vi "GettingStarted_RealSignals.vi"() -> ()   [LabVIEW 2009]
uses:
  <vilib>/imath/engines/lvmath2/RunTimeEngine/ErrorHandling/NIMS_Finalize Error.vi
  <vilib>/imath/engines/lvmath2/RunTimeEngine/Parser/MC_Version.vi
  <vilib>/imath/engines/lvmath2/RunTimeEngine/NodeEndStatement/NIMS_NodeEndStatement_Output.vi
  <instcachedir>/0/NIMS_NodeEndStatement_Output_53EC0D466D134D7ABD903AC30B43404B.lvgen/NIMS_NodeEndStatement_Output_53EC0D466D134D7ABD903AC30B43404B_001.vi
  <vilib>/imath/engines/lvmath2/RunTimeEngine/RangeToken/NIMS_Range.vi
  <instcachedir>/0/NIMS_Range_08574DECC23E450FAF0AC0BC39E6BEA7.lvgen/NIMS_Range_08574DECC23E450FAF0AC0BC39E6BEA7_001.vi
  <vilib>/imathl/engines/lvmath/Functions/Error Handling/Create Error.vi
  <vilib>/imath/engines/lvmath/Functions/Error Handling/MC_Error Cluster From Error Code.vi
  <vilib>/imath/engines/lvmath2/RunTimeEngine/BuiltInFunctions/rand/NIMS_rand(1,I32).vi
  <vilib>/imath/engines/lvmath/Functions/Error Handling/MergeErrorsWrapper.vi
  <vilib>/imath/engines/lvmath2/RunTimeEngine/BuiltInFunctions/abs/NIMS_abs(signed).vi
  <instcachedir>/0/NIMS_abs(signed)_C4FCB8E6058B49B797C7C8D53CA5F6EC.lvgen/NIMS_abs(signed)_C4FCB8E6058B49B797C7C8D53CA5F6EC_000.vi
  <vilib>/imath/engines/lvmath2/RunTimeEngine/BuiltInFunctions/fft/NIMS_fft(GV).vi
  <instcachedir>/0/NIMS_fft(GV)_4C6467FC22F84E4BA42517A07EF978B0.lvgen/NIMS_fft(GV)_4C6467FC22F84E4BA42517A07EF978B0_001.vi
  <vilib>/imath/engines/lvmath2/RunTimeEngine/ArithmeticOperatorToken/NIMS_ArithmeticOperator_plus.vi
  <instcachedir>/0/NIMS_ArithmeticOperator_plus_48B9519178ED42D7840F01273E784BFE.lvgen/NIMS_ArithmeticOperator_plus_48B9519178ED42D7840F01273E784BFE_000.vi
panel:
  in  "Spur Level (V)":dbl=0.001
  in  "Noise Level (V)":dbl(slide)=0.00024489795918367346 scale=0.0..0.001
  in  "Tab Control":T1(tab)=enum."Noise & Signal + Spur"
  out "x":dbl[](graph)=[0.0, 1.0, 2.0, 3.0, 4.0, 5.0, 6.0, 7.0, 8.0, 9.0, 10.0, 11.0, 12.0, 13.0, 14.0, 15.0, 16.0, 17.0, 18.0, 19.0, 20.0, 21.0, 22.0, 23.0, 24.0, 25.0, 26.0, 27.0, 28.0, 29.0, 30.0, 31.0, 32.0, 33.0, 34.0, 35.0, 36.0, 37.0, 38.0, 39.0, 40.0, 41.0, 42.0, 43.0, 44.0, 45.0, 46.0, 47.0, 48.0, 49.0, 50.0, 51.0, 52.0, 53.0, 54.0, 55.0, 56.0, 57.0, 58.0, 59.0, 60.0, 61.0, 62.0, 63.0]
  out "signal (Time Domain)":dbl[](graph)=[1.0, 0.9951847266721969, 0.9807852804032304, 0.9569403357322088, 0.9238795325112867, 0.881921264348355, 0.8314696123025452, 0.773010453362737, 0.7071067811865476, 0.6343932841636455, 0.5555702330196023, 0.4713967368259978, 0.38268343236508984, 0.29028467725446233, 0.19509032201612833, 0.09801714032956077, 6.123031769111886e-17, -0.09801714032956065, -0.1950903220161282, -0.29028467725446216, -0.3826834323650897, -0.4713967368259977, -0.555570233019602, -0.6343932841636454, -0.7071067811865475, -0.773010453362737, -0.8314696123025453, -0.8819212643483549, -0.9238795325112867, -0.9569403357322088, -0.9807852804032304, -0.9951847266721968, -1.0, -0.9951847266721969, -0.9807852804032304, -0.9569403357322089, -0.9238795325112868, -0.881921264348355, -0.8314696123025455, -0.7730104533627371, -0.7071067811865477, -0.6343932841636459, -0.5555702330196022, -0.47139673682599786, -0.38268343236509034, -0.29028467725446244, -0.19509032201612866, -0.09801714032956045, -1.836909530733566e-16, 0.09801714032956009, 0.1950903220161283, 0.29028467725446205, 0.38268343236509, 0.4713967368259976, 0.5555702330196018, 0.6343932841636456, 0.7071067811865474, 0.7730104533627367, 0.8314696123025452, 0.8819212643483548, 0.9238795325112865, 0.9569403357322088, 0.9807852804032303, 0.9951847266721969]
  out "noise (Time Domain)":dbl[](graph)=[0.00017345388847732183, 9.384721690440629e-05, 0.00021325506107333988, 9.033739461556139e-05, 8.225115957588394e-05, 0.00022899374260867145, 0.00017108200961533386, 4.3499454064839606e-05, 4.216960210159472e-05, 5.300855810985709e-05, 0.00022634691048571397, 4.142058298539253e-05, 0.00010698946173820982, 0.00017919168575125506, 0.000228746962935423, 0.00016811831847637424, 0.000149018054221302, 8.26228389545729e-05, 5.108267442002953e-05, 0.00022921494428844056, 0.00021666900139901673, 0.00018958850216650077, 6.182126932943757e-05, 0.0001013976231695041, 8.718964914935843e-05, 0.00013324340118243882, 0.0002384798798628175, 6.321954061707498e-05, 5.9741047834780797e-05, 4.5206442745249866e-05, 4.30637612234021e-05, 3.932217315793377e-05, 6.520083152831608e-05, 0.00023048966084202114, 3.048846374611175e-05, 4.528958373625526e-05, 4.425462708597921e-05, 0.00020517114908387817, 0.00014397299183518258, 0.00020960760994048083, 0.0001678937735573273, 0.00017945446738414523, 0.00014919763515730956, 0.00022121817515546554, 0.00010548017003027697, 0.00018691125297748206, 0.00014788947043336631, 5.466160312999556e-05, 1.0369681325846585e-05, 5.203831786508366e-05, 6.491243230331916e-05, 0.000236582660093371, 0.0001363150245849827, 4.065564633537551e-05, 7.924747061934878e-05, 0.00022262559485221323, 0.00011413358700753988, 3.354305722250164e-05, 0.00018280271967387516, 0.00022227396517330978, 0.0002219588013856892, 0.00021367238122965265, 2.8128510108291296e-05, 0.0002404575102916334]
  out "Signal+noise (Time Domain)":dbl[](graph)=[1.0001734538884772, 0.9952785738891013, 0.9809985354643038, 0.9570306731268244, 0.9239617836708626, 0.8821502580909637, 0.8316406943121606, 0.7730539528168018, 0.7071489507886491, 0.6344462927217553, 0.555796579930088, 0.4714381574089832, 0.38279042182682804, 0.2904638689402136, 0.19531906897906376, 0.09818525864803715, 0.00014901805422136324, -0.09793451749060607, -0.19503923934170816, -0.2900554623101737, -0.38246676336369073, -0.4712071483238312, -0.5555084117502725, -0.6342918865404759, -0.7070195915373981, -0.7728772099615545, -0.8312311324226825, -0.8818580448077379, -0.923819791463452, -0.9568951292894635, -0.980742216642007, -0.9951454044990389, -0.9999347991684717, -0.9949542370113549, -0.9807547919394843, -0.9568950461484726, -0.9238352778842008, -0.8817160931992711, -0.8313256393107102, -0.7728008457527966, -0.7069388874129904, -0.6342138296962618, -0.5554210353844449, -0.4711755186508424, -0.3825779521950601, -0.29009776600148496, -0.1949424325456953, -0.09796247872643045, 1.0369681325662894e-05, 0.09806917864742518, 0.19515523444843164, 0.2905212599145554, 0.382819747389675, 0.47143739247233296, 0.5556494804902212, 0.6346159097584978, 0.7072209147735549, 0.7730439964199591, 0.8316524150222191, 0.8821435383135281, 0.9241014913126722, 0.9571540081134384, 0.9808134089133386, 0.9954251841824886]
  out "Signal+noise (Frequency Domain)":dbl[](graph)=[-71.8050437272979, 0.00013005279351058333, -104.62327782338406, -87.75677400745508, -98.45829995492122, -98.02904136915537, -113.29022320138012, -95.68610292498795, -95.8079274126157, -100.83736132161248, -89.59002758572835, -93.46687419460775, -99.30705447635526, -91.94368354860872, -89.12999646522752, -96.28826637953654, -100.8795208279637, -92.91659234807581, -94.9930234903727, -94.71403092612485, -96.21706845313844, -97.98166741229112, -93.40743227426096, -96.68926525561577, -95.41577993723159, -94.80772868743333, -99.79729920228047, -100.11788143219786, -95.19912493512508, -96.12977454386336, -110.39055381850221, -94.26600936294412, -95.56391853930201, -94.26600936294412, -110.39055381850221, -96.12977454386336, -95.19912493512508, -100.11788143219786, -99.79729920228047, -94.80772868743333, -95.41577993723159, -96.68926525561577, -93.40743227426096, -97.98166741229112, -96.21706845313844, -94.71403092612485, -94.9930234903727, -92.91659234807581, -100.8795208279637, -96.28826637953654, -89.12999646522752, -91.94368354860872, -99.30705447635526, -93.46687419460775, -89.59002758572835, -100.83736132161248, -95.8079274126157, -95.68610292498795, -113.29022320138012, -98.02904136915537, -98.45829995492122, -87.75677400745508, -104.62327782338406, 0.00013005279351058333]
  out "Signal+noise+spur (Frequency Domain)":dbl[](graph)=[-71.80504372729874, 0.00013005279351058333, -104.62327782335703, -87.7567740074563, -98.45829995490946, -98.0290413691683, -113.29022320141122, -95.68610292496868, -95.80792741260979, -100.83736132158157, -59.74291088368047, -93.46687419459742, -99.30705447635629, -91.94368354862048, -89.1299964652258, -59.89611367928067, -100.87952082796554, -92.91659234808257, -94.99302349036492, -94.71403092612033, -96.21706845313736, -97.98166741230378, -93.40743227426019, -96.68926525560991, -95.41577993723067, -94.80772868742562, -99.79729920228023, -100.11788143219661, -95.1991249351243, -96.12977454386142, -110.39055381848462, -94.26600936293949, -95.56391853929411, -94.26600936293949, -110.39055381848462, -96.12977454386142, -95.1991249351243, -100.11788143219661, -99.79729920228023, -94.80772868742562, -95.41577993723067, -96.68926525560991, -93.40743227426019, -97.98166741230378, -96.21706845313736, -94.71403092612033, -94.99302349036492, -92.91659234808257, -100.87952082796554, -59.89611367928067, -89.1299964652258, -91.94368354862048, -99.30705447635629, -93.46687419459742, -59.74291088368047, -100.83736132158157, -95.80792741260979, -95.68610292496868, -113.29022320141122, -98.0290413691683, -98.45829995490946, -87.7567740074563, -104.62327782335703, 0.00013005279351058333]
  out "Signal+noise+spur (Time Domain)":dbl[](graph)=[1.002173453888477, 0.9959321612624504, 0.9796350667515354, 0.9557596031691667, 0.9241785564221873, 0.8828167451498058, 0.8317331042323693, 0.7732510291449407, 0.7078560575698357, 0.6343878335628156, 0.5543171301645572, 0.47036114582261873, 0.3838802120403797, 0.292401594556349, 0.19550666208941272, 0.09663450368834536, -0.0008509819457786394, -0.09749490299695349, -0.19446146558732696, -0.29003161736550265, -0.38214234001486924, -0.470520317381499, -0.5558767210497643, -0.6358963666061411, -0.7077266983185847, -0.7714113470650884, -0.8294757832778688, -0.8821343512225477, -0.9254507777771498, -0.9575856298926123, -0.9801441147939689, -0.9946878514063489, -0.9999347991684717, -0.9944966839186649, -0.9801566900914462, -0.9575855467516214, -0.9254662641978987, -0.8819923996140809, -0.8295702901658965, -0.7713349828563305, -0.707645994194177, -0.6358183097619271, -0.5557893446839366, -0.47048868770851016, -0.38225352884623864, -0.2900739210568139, -0.1943646587913141, -0.09752286423277787, -0.000989630318674336, 0.09651842368773338, 0.19534282755878057, 0.29245898553069083, 0.38390953760322666, 0.4703603808859685, 0.5541700307246903, 0.634557450599558, 0.7079280215547414, 0.7732410727480981, 0.8317448249424279, 0.8828100253723702, 0.9243182640639969, 0.9558829381557807, 0.9794499402005702, 0.9960787715558377]
  in  "np":dbl=64.0 caption="Number of Points"
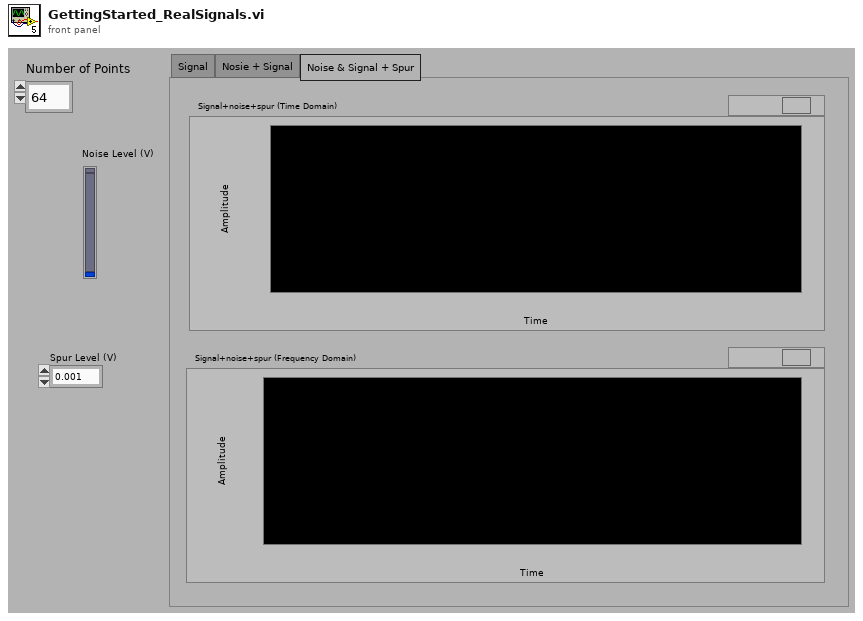
[diagram p1: front panel]
types:
  T1 = enum32{"Signal", "Nosie + Signal", "Noise & Signal + Spur"}
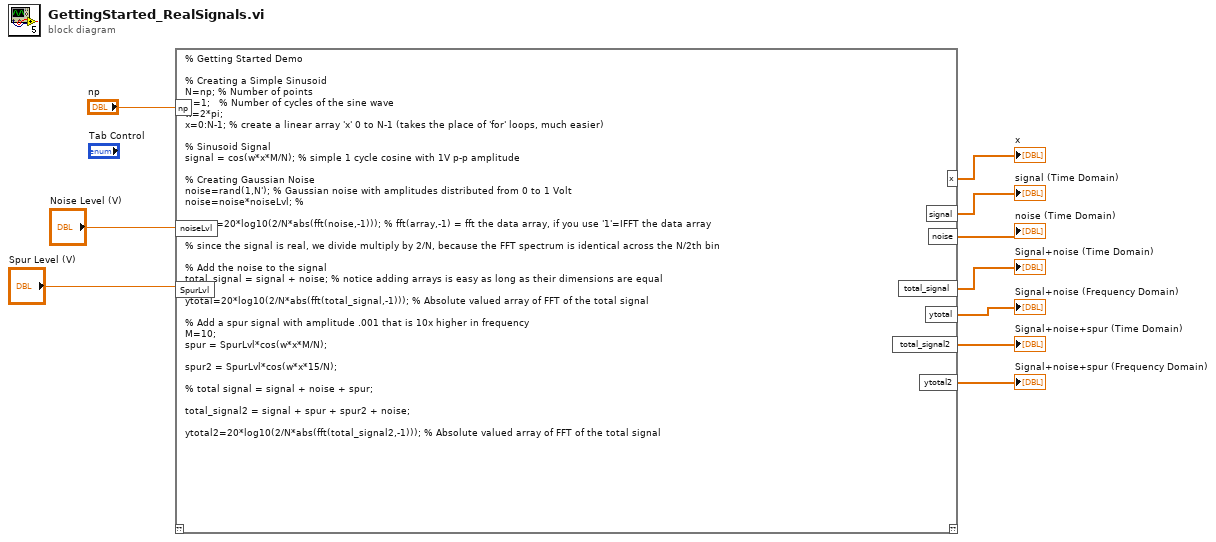
[diagram p0: block diagram]
diagram:
  n1 = mathscript code="% Getting Started Demo\n\n% Creating a Simple Sinusoid\nN=np; % Number of points\nM=1;   % Number of cycles of the sine wave\nw=2*pi; \nx=0:N-1; % create a linear array 'x' 0 to N-1 (takes the place of 'for' loops, much easier)\n\n% Sinusoid Signal\nsignal = cos(w*x*M/N); % simple 1 cycle cosine with 1V p-p amplitude\n\n% Creating Gaussian Noise\nnoise=rand(1,N'); % Gaussian noise with amplitudes distributed from 0 to 1 Volt\nnoise=noise*noiseLvl; % \n\nynoise=20*log10(2/N*abs(fft(noise,-1))); % fft(array,-1) = fft the data array, if you use '1'=IFFT the data array\n\n% since the signal is real, we divide multiply by 2/N, because the FFT spectrum is identical across the N/2th bin\n\n% Add the noise to the signal\ntotal_signal = signal + noise; % notice adding arrays is easy as long as their dimensions are equal\n\nytotal=20*log10(2/N*abs(fft(total_signal,-1))); % Absolute valued array of FFT of the total signal \n\n% Add a spur signal with amplitude .001 that is 10x higher in frequency\nM=10; \nspur = SpurLvl*cos(w*x*M/N);\n\nspur2 = SpurLvl*cos(w*x*15/N);\n\n% total signal = signal + noise + spur;\n\ntotal_signal2 = signal + spur + spur2 + noise;\n\nytotal2=20*log10(2/N*abs(fft(total_signal2,-1))); % Absolute valued array of FFT of the total signal"("np"="np", "noiseLvl"="Noise Level (V)", "SpurLvl"="Spur Level (V)") -> ("noise"=→"noise (Time Domain)":dbl[], "ytotal"=→"Signal+noise (Frequency Domain)":dbl[], "x"=→"x":dbl[], "signal"=→"signal (Time Domain)":dbl[], "total_signal"=→"Signal+noise (Time Domain)":dbl[], "total_signal2"=→"Signal+noise+spur (Time Domain)":dbl[], "ytotal2"=→"Signal+noise+spur (Frequency Domain)":dbl[])  [unwired: 1 in, 1 out]
